vi "FTW-Example-AddEventLoggerToLegacyCode.vi"() -> ()   [LabVIEW 2013]
uses:
  Actor/src/EventLogger/FTW-Logger.lvclass
  Actor/src/Ether/FTW-Ether.lvclass
panel:
  out "error out":errorcluster
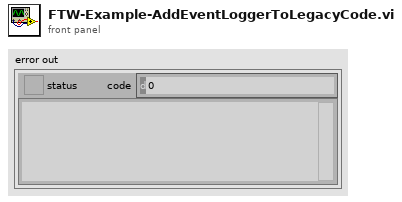
[diagram p1: front panel]
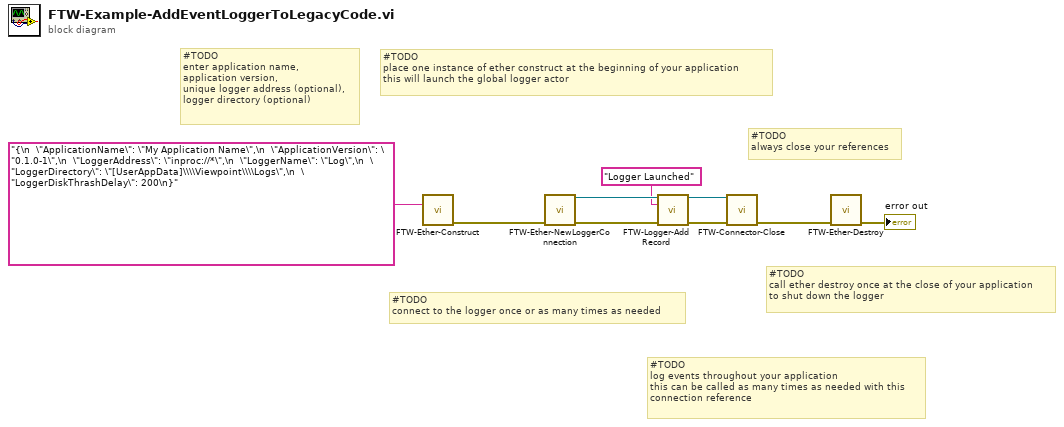
[diagram p0: block diagram]
diagram:
  # "#TODO\ncall ether destroy once at the close of your application\nto shut down the logger"
  # "#TODO\nalways close your references"
  # "#TODO\nlog events throughout your application\nthis can be called as many times as needed with this\nconnection reference"
  # "#TODO\nconnect to the logger once or as many times as needed"
  # "#TODO\nplace one instance of ether construct at the beginning of your application\nthis will launch the global logger actor"
  # "#TODO\nenter application name,\napplication version,\nunique logger address (optional),\nlogger directory (optional)"
  n1 = call "FTW-Ether-Construct.vi"("FTW Ether Configuration"="{\n  \"ApplicationName\": \"My Application Name\",\n  \"ApplicationVersion\": \"0.1.0-1\",\n  \"LoggerAddress\": \"inproc://*\",\n  \"LoggerName\": \"Log\",\n  \"LoggerDirectory\": \"[UserAppData]\\\\Viewpoint\\\\Logs\",\n  \"LoggerDiskThrashDelay\": 200\n}") -> ("error out"=w4:errorcluster)  [unwired: 14 in]
  n2 = call "FTW-Ether-NewLoggerConnection.vi"("error in"=w4) -> ("Event Logger Connection"=w9:refnum<class "FTW-Logger.lvclass">, "error out"=w8:errorcluster)  [unwired: 13 in]
  n3 = call "FTW-Logger-AddRecord.vi"("FTW Logger Connector"=w9, "Event Type"="Logger Launched", "error in"=w8) -> ("FTW Logger Connector out"=w5:refnum<class "FTW-Logger.lvclass">, "error out"=w7:errorcluster)  [unwired: 10 in, 1 out]
  n4 = call-dynamic "FTW-Connector-Close.vi"("FTW Actor Connector"=w5, "error in"=w7) -> ("error out"=w2:errorcluster)  [unwired: 13 in]
  n5 = call "FTW-Ether-Destroy.vi"("error in"=w2) -> ("error out"=→"error out":errorcluster)  [unwired: 14 in]
